vi "Set Source Value.vi"(8 "error in (no error)":errorcluster, 9 "Source Value Units":T1, 10 "Source Value":dbl, 11 "Keithley 2400 in":refnum<class "Keithley 2400.lvclass">) -> (0 "error out":errorcluster, 3 "Keithley 2400 out":refnum<class "Keithley 2400.lvclass">)   [LabVIEW 2011, in "Keithley 2400.lvclass"]
uses:
  Keithley 2400.lvclass
  Power Supply/Source Units.ctl
  Power Supply/Source Mode.ctl
  Keithley 2400.lvclass/Keithley 2400.ctl
  <instrlib>/Keithley 24XX/Keithley 24XX.lvlib
  Power Supply/Power Supply.lvclass
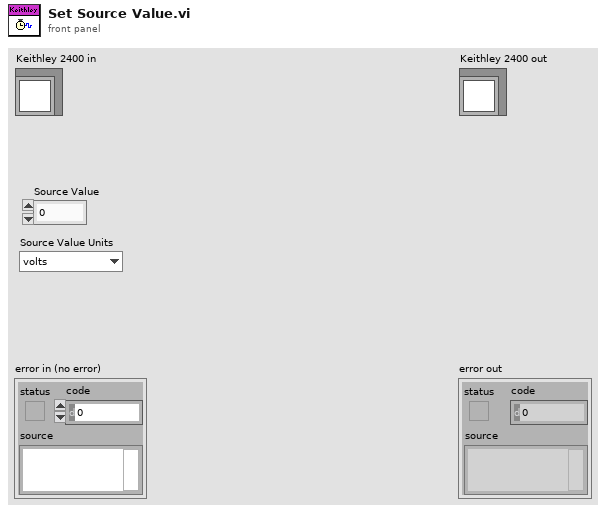
[diagram p1: front panel]
types:
  T1 = typedef "Power Supply.lvclass/Source Units.ctl" = enum16{"volts", "millivolts", "microvolts", "amps", "milliamps", "microamps", "nanoamps"}
  T2 = typedef "Power Supply.lvclass/Source Mode.ctl" = enum16{"Volts", "Current"}
  T3 = typedef "Power Supply.lvclass/Protection Limits.ctl" = cluster{"Voltage Limit":dbl, "Voltage Limit Units":T4, "Current Limit":dbl, "Current Limit Units":T5, "Voltage Trip/Cmpl":dbl, "Voltage Trip/Cmpl Units":T4, "Current Trip/Cmpl":dbl, "Current Trip/Cmpl Units":T5}
  T4 = typedef "Power Supply.lvclass/Voltage Units.ctl" = enum16{"volts", "millivolts", "microvolts"}
  T5 = typedef "Power Supply.lvclass/Current Units.ctl" = enum16{"amps", "milliamps", "microamps", "nanoamps"}
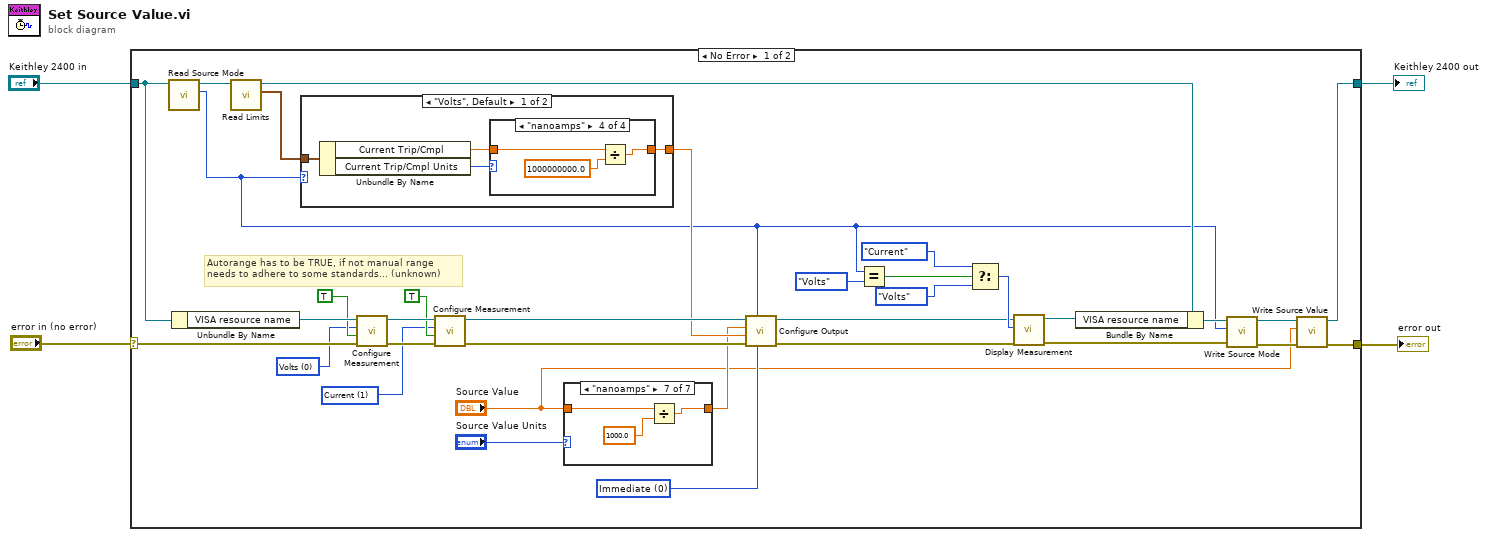
[diagram p0: block diagram]
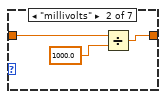
[diagram p3: hidden frame]
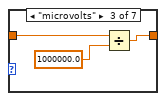
[diagram p4: hidden frame]
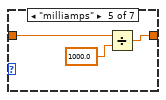
[diagram p6: hidden frame]
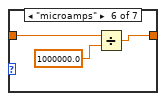
[diagram p7: hidden frame]
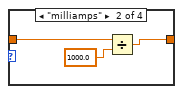
[diagram p9: hidden frame]
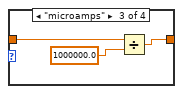
[diagram p10: hidden frame]
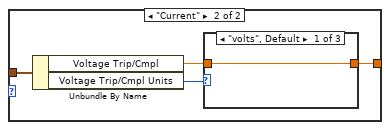
[diagram p11: hidden frame]
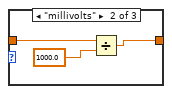
[diagram p12: hidden frame]
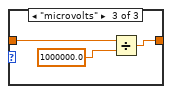
[diagram p13: hidden frame]
diagram:
  n1 = case shown="No Error" "error in (no error)" {
    selector: "error in (no error)" -> [w37 w82]
    tunnel: [w8 w82] -> w3
    tunnel: [w7 w81] -> w1
    tunnel: "Keithley 2400 in" -> [w12 w81]
    frame No Error {
      w27 = u16 0 items=["Immediate", "Triggered"] ("Output Type  (0: Immediate)")
      w30 = u16 1 items=["Volts", "Current", "Resistance"] ("Function (0: Volts)")
      w31 = u16 0 items=["Volts", "Current", "Resistance"] ("Function (0: Volts)")
      # "Autorange has to be TRUE, if not manual range\nneeds to adhere to some standards... (unknown)"
      n2 = call-dynamic "Read Source Mode.vi"("Power Supply in"=w12) -> ("Source Mode"=w10:T2, "Power Supply out"=w11:refnum<class "Keithley 2400.lvclass">)  [unwired: 8 in, 1 out]
      n3 = Unbundle By Name(w12) -> ("VISA resource name"=w38:refnum<visa-resource-name>)
      n4 = call-dynamic "Read Limits.vi"("Power Supply in"=w11) -> ("Protection Limits"=w16:T3, "Power Supply out"=w17:refnum<class "Keithley 2400.lvclass">)  [unwired: 8 in, 1 out]
      n5 = case shown="\"Volts\", Default" w10 {
        tunnel: w16 -> [w59 w73]
        tunnel: [w56 w70] -> w15
        frame "Volts", Default {
          n6 = Unbundle By Name(w59) -> ("Current Trip/Cmpl"=w57:dbl, "Current Trip/Cmpl Units"=w58:T5)
          n7 = case shown="\"nanoamps\"" w58 {
            tunnel: w57 -> [w60 w63 w66 w69]
            tunnel: [w60 w62 w64 w67] -> w56
            frame "amps", Default {
            }
            frame "milliamps" {
              n8 = Divide(x=w63, y=1000.0) -> (x/y=w62:dbl)
            }
            frame "microamps" {
              n9 = Divide(x=w66, y=1000000.0) -> (x/y=w64:dbl)
            }
            frame "nanoamps" {
              n10 = Divide(x=w69, y=1000000000.0) -> (x/y=w67:dbl)
            }
          }
        }
        frame "Current" {
          n11 = Unbundle By Name(w73) -> ("Voltage Trip/Cmpl"=w71:dbl, "Voltage Trip/Cmpl Units"=w72:T4)
          n12 = case shown="\"volts\", Default" w72 {
            tunnel: w71 -> [w74 w77 w80]
            tunnel: [w74 w75 w78] -> w70
            frame "volts", Default {
            }
            frame "millivolts" {
              n13 = Divide(x=w77, y=1000.0) -> (x/y=w75:dbl)
            }
            frame "microvolts" {
              n14 = Divide(x=w80, y=1000000.0) -> (x/y=w78:dbl)
            }
          }
        }
      }
      n15 = call <instrlib>:"Configure Measurement.vi"("error in (no error)"=w37, "Enable Auto Range (T:Enable)"=TRUE, "Function (0: Volts)"=w31, "VISA resource name"=w38) -> ("error out"=w34:errorcluster, "VISA resource name out"=w33:refnum<visa-resource-name>)  [unwired: 6 in]
      n16 = call <instrlib>:"Configure Measurement.vi"("error in (no error)"=w34, "Enable Auto Range (T:Enable)"=TRUE, "Function (0: Volts)"=w30, "VISA resource name"=w33) -> ("error out"=w28:errorcluster, "VISA resource name out"=w29:refnum<visa-resource-name>)  [unwired: 6 in]
      n17 = case shown="\"nanoamps\"" "Source Value Units" {
        tunnel: "Source Value" -> [w39 w41 w44 w46 w48 w51 w54]
        tunnel: [w39 w40 w43 w46 w47 w50 w53] -> w13
        frame "volts", Default {
        }
        frame "millivolts" {
          n18 = Divide(x=w41, y=1000.0) -> (x/y=w40:dbl)
        }
        frame "microvolts" {
          n19 = Divide(x=w44, y=1000000.0) -> (x/y=w43:dbl)
        }
        frame "amps" {
        }
        frame "milliamps" {
          n20 = Divide(x=w48, y=1000.0) -> (x/y=w47:dbl)
        }
        frame "microamps" {
          n21 = Divide(x=w51, y=1000000.0) -> (x/y=w50:dbl)
        }
        frame "nanoamps" {
          n22 = Divide(x=w54, y=1000.0) -> (x/y=w53:dbl)
        }
      }
      n23 = call <instrlib>:"Configure Output.vi"("Output Type  (0: Immediate)"=w27, "Source Mode  (0: Voltage)"=w10, "error in (no error)"=w28, "Compliance  Level (0.1)"=w15, "Output Level (0)"=w13, "VISA resource name"=w29) -> ("error out"=w21:errorcluster, "VISA resource name out"=w19:refnum<visa-resource-name>)  [unwired: 4 in]
      n24 = Equal?(x=w10, y=Source_Mode."Volts") -> (x = y?=w25:bool)
      n25 = Select(t=Source_Mode."Current" ("y"), s=w25, f=Source_Mode."Volts" ("y")) -> (s? t:f=w22:T2)
      n26 = call <instrlib>:"Display Measurement.vi"("error in (no error)"=w21, "Displayed Measurement (0: Voltage)"=w22, "VISA resource name"=w19) -> ("error out"=w20:errorcluster, "VISA resource name out"=w18:refnum<visa-resource-name>)  [unwired: 7 in]
      n27 = Bundle By Name(cluster=w17, "VISA resource name"=w18) -> (w36:refnum<class "Keithley 2400.lvclass">)
      n28 = call-dynamic "Write Source Mode.vi"("error in (no error)"=w20, "Source Mode"=w10, "Power Supply in"=w36) -> ("error out"=w9:errorcluster, "Power Supply out"=w6:refnum<class "Keithley 2400.lvclass">)  [unwired: 7 in]
      n29 = call-dynamic "Write Source Value.vi"("error in (no error)"=w9, "Source Value"="Source Value", "Power Supply in"=w6) -> ("error out"=w8:errorcluster, "Power Supply out"=w7:refnum<class "Keithley 2400.lvclass">)  [unwired: 7 in]
    }
    frame Error {
    }
  }
  "error out" <- w3
  "Keithley 2400 out" <- w1
